vi "Add Compensator Flow.vi"(8 "error in (no error)":errorcluster, 10 "Compensator Parameter Name (flow_rate_compensator)":string="flow_rate_compensator", 11 "New Parameters (percents)":T1) -> (0 "error out":errorcluster, 3 "New Parameters (percents) out":T1)   [LabVIEW 2020, in "Deep Reaction Optimizer Control Panel.lvlib" / "Instrument Manager.lvlib"]
uses:
  Instrument Manager.lvlib
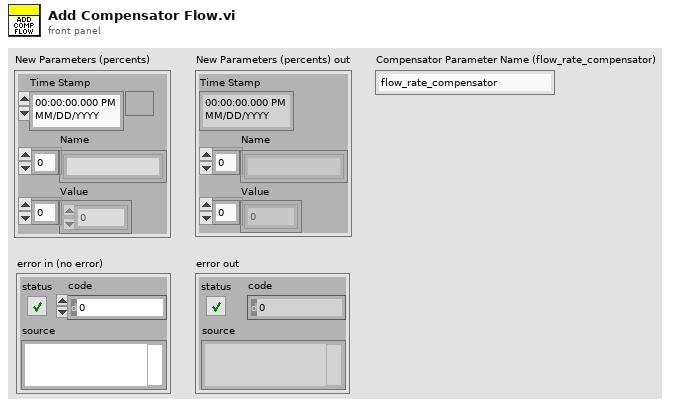
[diagram p1: front panel]
types:
  T1 = cluster{"Time Stamp":timestamp, "Name":string[], "Value":dbl[]}
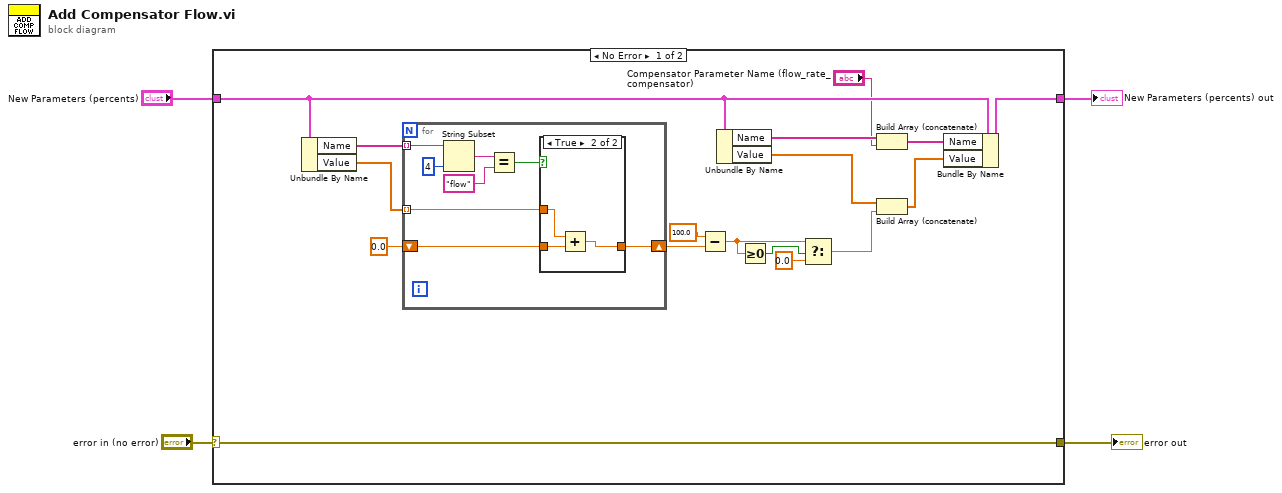
[diagram p0: block diagram]
diagram:
  n1 = case shown="No Error" "error in (no error)" {
    selector: "error in (no error)" -> [w21 w34]
    tunnel: "New Parameters (percents)" -> [w18 w35]
    tunnel: [w11 w35] -> w1
    tunnel: [w21 w34] -> w3
    frame No Error {
      n2 = Unbundle By Name(w18) -> ("Name"=w20:string[], "Value"=w15:dbl[])
      n3 = for {
        tunnel: w20 -> [w29] mode=indexing
        shift-right: [w24] -> w17
        shift-left: 0.0 -> [w23]
        tunnel: w15 -> [w22] mode=indexing
        n4 = String Subset(string=w29, length (rest)=4 ("length (rest)")) -> (substring=w27:string)  [unwired: 1 in]
        n5 = Equal?(x=w27, y="flow") -> (x = y?=w25:bool)
        n6 = case shown="True" w25 {
          tunnel: w22 -> [_ w31]
          tunnel: [w30 w33] -> w24
          tunnel: w23 -> [w30 w32]
          frame False {
          }
          frame True {
            n7 = Add(x=w31, y=w32) -> (x+y=w33:dbl)
          }
        }
      }
      n8 = Subtract(x=100.0, y=w17) -> (x-y=w6:dbl)
      n9 = Unbundle By Name(w18) -> ("Name"=w14:string[], "Value"=w12:dbl[])
      n10 = Greater Or Equal To 0?(x=w6) -> (x >= 0?=w5:bool)
      n11 = Select(t=w6, s=w5, f=0.0) -> (s? t:f=w8:dbl)
      n12 = Build Array (concatenate)(w14, "Compensator Parameter Name (flow_rate_compensator)") -> (w10:string[])
      n13 = Build Array (concatenate)(w12, w8) -> (w9:dbl[])
      n14 = Bundle By Name(cluster=w18, "Name"=w10, "Value"=w9) -> (w11:T1)
    }
    frame Error {
    }
  }
  "error out" <- w3
  "New Parameters (percents) out" <- w1
